vi "SetSession.vi"(8 "error in (no error)":errorcluster, 10 "Session":path=path "Z:/users/Manolis/Labview/Water Conditioning/sessions_Win7.dsn", 11 "Database in":refnum<class "Database.lvclass">) -> (0 "error out":errorcluster, 3 "Database out":refnum<class "Database.lvclass">)   [LabVIEW 2014, in "Database.lvclass"]
uses:
  Database.lvclass
  Database.lvclass/Database.ctl
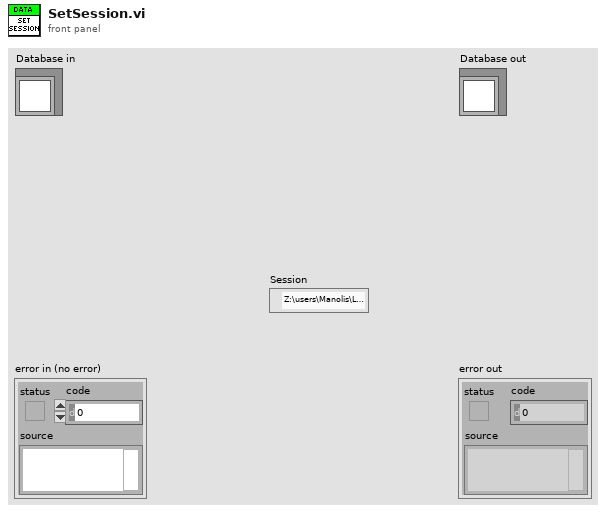
[diagram p1: front panel]
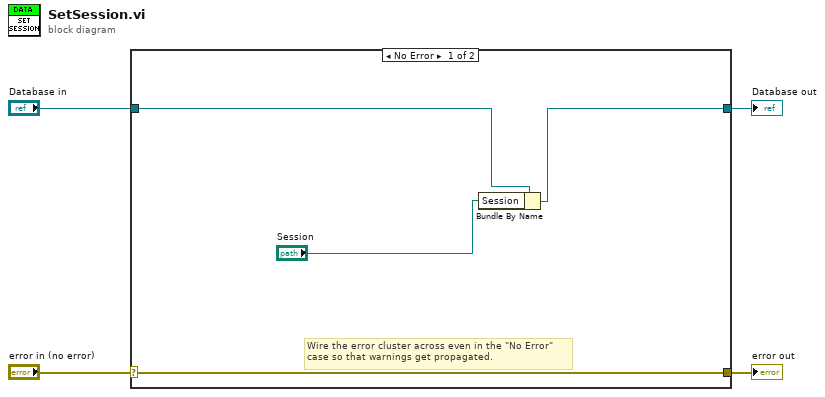
[diagram p0: block diagram]
diagram:
  n1 = case shown="No Error" "error in (no error)" {
    selector: "error in (no error)" -> [w8 w10]
    tunnel: [w8 w10] -> w3
    tunnel: [w5 w9] -> w1
    tunnel: "Database in" -> [w7 w9]
    frame No Error {
      # "Wire the error cluster across even in the \"No Error\"\ncase so that warnings get propagated."
      n2 = Bundle By Name(cluster=w7, "Session"="Session") -> (w5:refnum<class "Database.lvclass">)
    }
    frame Error {
    }
  }
  "error out" <- w3
  "Database out" <- w1
